vi "WaveformGraph.vi"() -> ()   [LabVIEW 2012]
panel:
  out "Waveform Graph":dbl[](graph)
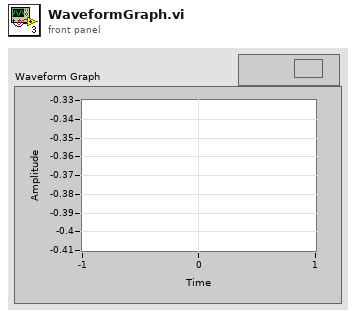
[diagram p1: front panel]
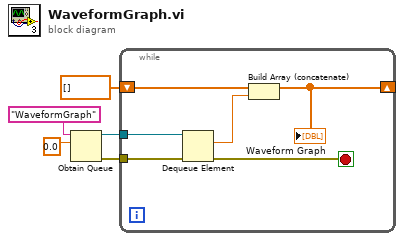
[diagram p0: block diagram]
diagram:
  n1 = Obtain Queue(name (unnamed)="WaveformGraph", element data type=0.0 ("Waveform Chart")) -> (queue out=w2:refnum<queue>, error out=w5:errorcluster)  [unwired: 3 in, 1 out]
  n2 = while {
    tunnel: w5 -> [w11]
    tunnel: w2 -> [w10]
    shift-right: [w7] -> _
    shift-left: dbl[] [] -> [w6]
    stop <- w9 stop-if-true
    n3 = Dequeue Element(queue=w10, error in (no error)=w11) -> (element=w8:dbl, error out=w9:errorcluster)  [unwired: 1 in, 2 out]
    n4 = Build Array (concatenate)(w6, w8) -> (w7:dbl[])
    "Waveform Graph" <- w7
  }
